vi "check multiple instances.vi"(7 "nb instances":i16=7, 8 "array elements in":bool[](array[boolean]), 11 "new element":bool) -> (0 "array elements out":bool[](array[boolean]), 3 "out":bool)   [LabVIEW 2021]
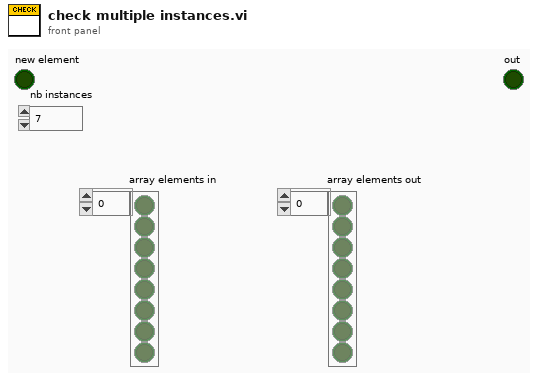
[diagram p1: front panel]
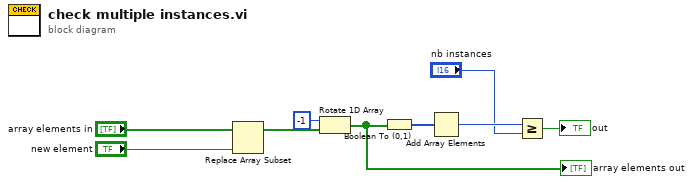
[diagram p0: block diagram]
diagram:
  n1 = Replace Array Subset(array="array elements in", new element="new element") -> (w7:bool[])  [unwired: 1 in]
  n2 = Rotate 1D Array(1:w7, 2:-1 ("n")) -> (0:w1:bool[])
  "array elements out" <- w1
  n3 = Boolean To (0,1)(Boolean=w1) -> (0, 1=w5:i16[])
  n4 = Add Array Elements(numeric array=w5) -> (sum=w4:i16)
  n5 = Greater Or Equal?(x=w4, y="nb instances") -> (x >= y?=→"out":bool)
